vi "Created.vi"(8 "Created Alias":string, 9 "Priority?":bool, 10 "Msg Strategy":refnum<class "Msg Strategy.lvclass">, 11 "jettl in":refnum<class "jettl.lvclass">) -> (3 "jettl out":refnum<class "jettl.lvclass">)   [LabVIEW 2021, in "jettl.lvlib" / "jettl.lvclass"]
uses:
  jettl.lvclass
  Msg Strategy/Msg Strategy.lvclass
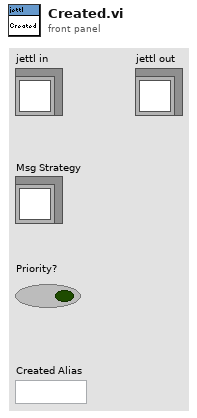
[diagram p1: front panel]
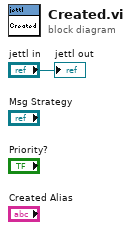
[diagram p0: block diagram]
diagram:
  "jettl out" <- "jettl in"
